vi "Write-Sync-with-TypeResolving-Sensata.vi"() -> ()   [LabVIEW 2020]
doc: "ADS synchronous write example using preconfigured blocks. \n\nThe client writes data synchronously and does wait for the respose from server."
uses:
  <userlib>/Beckhoff-LabVIEW-Interface/_DependsOn/TypeDefs/Low-Levels/Symbol Interface Mode.ctl
  <userlib>/Beckhoff-LabVIEW-Interface/_DependsOn/With TypeResolving/Write Sync Single TypeResolved.vi
panel:
  in  "sVar":string="TF3710"
  out "Has Matched?":bool
  in  "Symbol file path":path
  out "Write Status":bool
  # "The example starts with retrieving an\nADS Symbol. The symbol can be selected:\n- Using Symbol file in symbol file path\n- Using Symbol Interface (UI), which is opened automatically if file path is empty.\n\nThe example writes , only once, a string value synchronously to a string variable located in TwinCAT3. Since the  call is synchronous, the example waits for a timeout for an ADS response.\n\nThe example uses TypeResolver to check whether the selected ADS Symbol is of type String or not.\n\nCheck Write status and bHasMached if write has succeeded."
  # "Note: This example is only an illustration of all possible ways how this Product can be used."
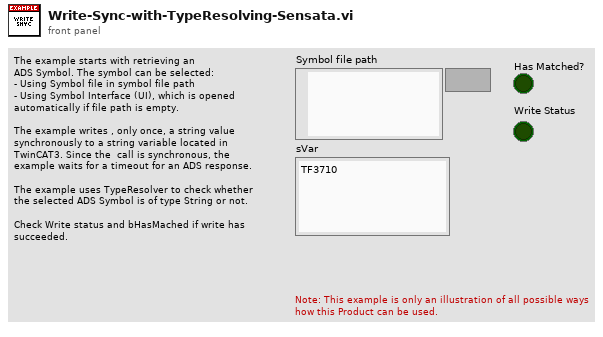
[diagram p1: front panel]
types:
  T1 = cluster{"nVar1":i16, "nVar2":u32, "sVar3":string[]}
  T2 = typedef "Symbol Interface Mode.ctl" = enum16{"Read Only", "Write Only", "Read & Write"}
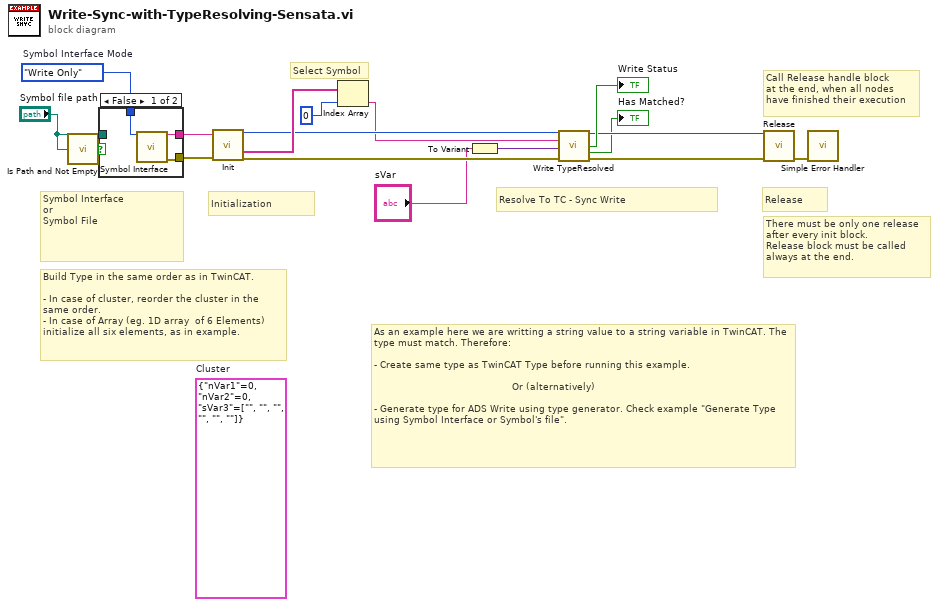
[diagram p0: block diagram]
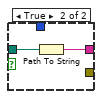
[diagram p2: hidden frame]
diagram:
  (unwired) T1 {"nVar1"=0, "nVar2"=0, "sVar3"=["", "", "", "", "", ""]}  # Cluster
  w2 = Symbol_Interface_Mode."Write Only"  # Symbol Interface Mode
  # "As an example here we are writting a string value to a string variable in TwinCAT. The type must match. Therefore:\n\n- Create same type as TwinCAT Type before running this example. \n                                              \n                                              Or (alternatively)\n\n- Generate type for ADS Write using type generator. Check example \"Generate Type using Symbol Interface or Symbol's file\"."
  # "Build Type in the same order as in TwinCAT.\n\n- In case of cluster, reorder the cluster in the\nsame order.\n- In case of Array (eg. 1D array  of 6 Elements) \ninitialize all six elements, as in example."
  # "Symbol Interface\nor\nSymbol File"
  # "Resolve To TC - Sync Write"
  # "Call Release handle block\nat the end, when all nodes\nhave finished their execution"
  # "There must be only one release\nafter every init block.\nRelease block must be called\nalways at the end."
  # "Select Symbol"
  # "Release"
  # "Initialization"
  n1 = call <vilib>:"Is Path and Not Empty.vi"("path"="Symbol file path") -> ("Is Path and Not Empty?"=w3:bool)  [unwired: 4 in]
  n2 = case shown="False" w3 {
    tunnel: [w20 w22] -> w4
    tunnel: "Symbol file path" -> [_ w21]
    tunnel: [w19 _] -> w5
    tunnel: w2 -> [w18 _]
    frame False {
      n3 = call <userlib>:"Symbol Interface.vi"("Symbol Interface Mode"=w18) -> ("PortInfo"=w20:string, "error out"=w19:errorcluster)  [unwired: 13 in]
    }
    frame True {
      n4 = Path To String(path=w21) -> (string=w22:string)
    }
  }
  n5 = call <userlib>:"Init.vi"("XMLDescription"=w4, "error in (no error)"=w5) -> ("Handle"=w15:u32, "WriteGrpSymbols"=w16:string[], "error out"=w13:errorcluster)  [unwired: 9 in, 2 out]
  n6 = Index Array(array=w16, index=0) -> (element=w14:string)
  n7 = To Variant(anything="sVar") -> (Variant=w12:variant)
  n8 = call-poly <userlib>:"Write TypeResolved.vi"("Handle"=w15, "SymbolName"=w14, "WData"=w12, "error constant"=w13) -> ("Handle"=w9:u32, "Write Status?"=→"Write Status":bool, "Has Matched?"=→"Has Matched?":bool, "error out"=w10:errorcluster)  [unwired: 8 in]
  n9 = call <userlib>:"Release.vi"("Handle"=w9, "error in (no error)"=w10) -> ("error out"=w1:errorcluster)  [unwired: 13 in]
  n10 = call <vilib>:"Simple Error Handler.vi"("error in (no error)"=w1) -> ()  [unwired: 4 in, 5 out]
